vi "sell.vi"(8 "error in (no error)":errorcluster, 11 "Stock in":refnum<class "Stock.lvclass">) -> (0 "error out":errorcluster, 3 "Stock out":refnum<class "Stock.lvclass">)   [LabVIEW 2018, in "Stock.lvclass"]
uses:
  Stock.lvclass
  ConsoleOut/Print Options.ctl
  Stock.lvclass/Stock.ctl
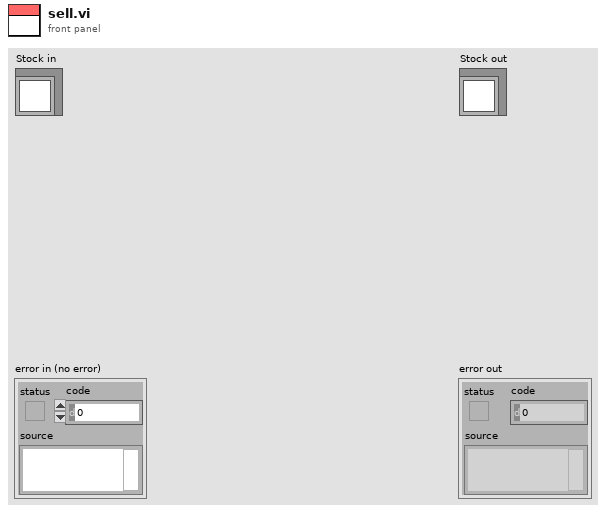
[diagram p1: front panel]
types:
  T1 = typedef "Print Options.ctl" = enum16{"Create", "Get Reference", "Print", "Print Header", "Close"}
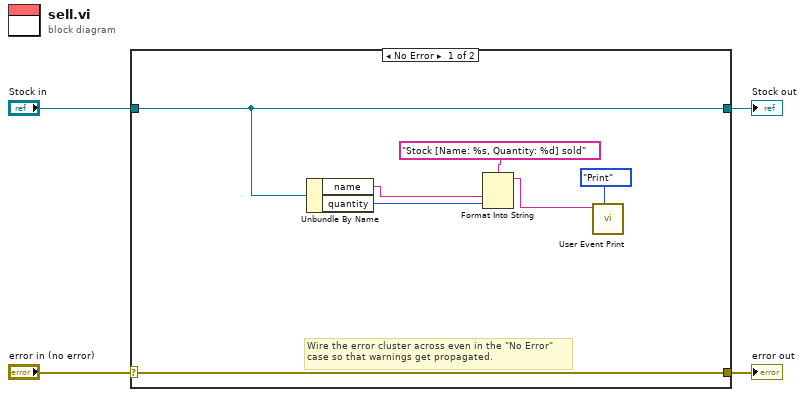
[diagram p0: block diagram]
diagram:
  n1 = case shown="No Error" "error in (no error)" {
    selector: "error in (no error)" -> [w11 w13]
    tunnel: [w11 w13] -> w3
    tunnel: [w7 w12] -> w1
    tunnel: "Stock in" -> [w7 w12]
    frame No Error {
      # "Wire the error cluster across even in the \"No Error\"\ncase so that warnings get propagated."
      n2 = Unbundle By Name(w7) -> ("name"=w9:string, "quantity"=w8:u8)
      n3 = Format Into String(format string="Stock [Name: %s, Quantity: %d] sold", w9, w8) -> (resulting string=w6:string)  [unwired: 2 in, 1 out]
      n4 = call "User Event Print.vi"("Options"=Print_Options."Print", "String to Print"=w6) -> ()  [unwired: 8 in, 2 out]
    }
    frame Error {
    }
  }
  "error out" <- w3
  "Stock out" <- w1
